vi "Uninit.vi"(11 "UI Template in":refnum<class "Root.lvclass">) -> (3 "UI Template out":refnum<class "Root.lvclass">)   [LabVIEW 2025, in "Root.lvlib" / "Root.lvclass"]
doc: "This method is the inverse of the Pre Launch Init.vi. This method is called unconditionally at the end of an actor's lifetime, even if there was an error in Pre Launch Init.vi. Note that the self Enqueuer for the actor is already invalid by the time this VI executes: within this method, the actor may send messages to its caller but not to itself. This method executes before Last Ack is sent.\n\nThis method neither receives nor produces an error cluster. It is designed to provide an unconditional release of acquired resources. Any error raised during release is considered to be irrelevant to the actor's lifetime. If the actor truly needs to report some error status, it may send a message to caller or include information within itself that callers can examine when handling Last Ack."
uses:
  Root.lvclass
  <vilib>/ActorFramework/Actor/Actor.lvclass
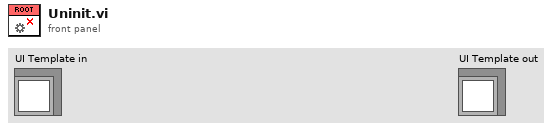
[diagram p1: front panel]
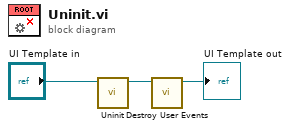
[diagram p0: block diagram]
diagram:
  n1 = call-parent "Uninit.vi"("Actor in"="UI Template in") -> ("Actor out"=w1:refnum<class "Root.lvclass">)  [unwired: 10 in]
  n2 = call "Destroy User Events.vi"("UI Template in"=w1) -> ("UI Template out"=→"UI Template out":refnum<class "Root.lvclass">)  [unwired: 10 in]
